vi "DMMP_GetBaselinePick.vi"(3 "Input DMMP":refnum<class "DMMP.lvclass">) -> (0 "Baseline Pick":enum16{"Manual", "Auto"}(ring), 1 "Output DMMP":refnum<class "DMMP.lvclass">)   [LabVIEW 2014, in "DMMP.lvclass"]
uses:
  DMMP.lvclass
  DMMP.lvclass/DMMP.ctl
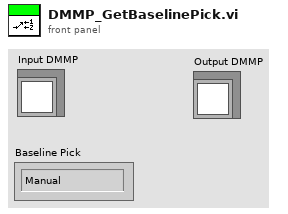
[diagram p1: front panel]
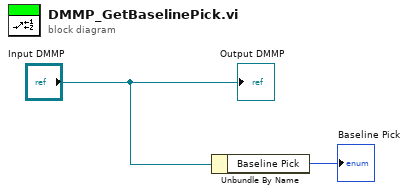
[diagram p0: block diagram]
diagram:
  n1 = Unbundle By Name("Input DMMP") -> ("Baseline Pick"=→"Baseline Pick":enum16{"Manual", "Auto"})
  "Output DMMP" <- "Input DMMP"
